vi "Get Events.vi"(11 "Create Sensor View in":refnum<class "Create Sensor View.lvclass">) -> (2 "Events":T1, 3 "Create Sensor View out":refnum<class "Create Sensor View.lvclass">)   [LabVIEW 2013, in "Create Sensor View.lvlib" / "Create Sensor View.lvclass"]
uses:
  Create Sensor View.lvclass
  Typedef/Events.ctl
  Create Sensor View.lvclass/Create Sensor View.ctl
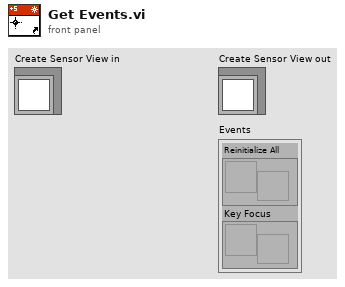
[diagram p1: front panel]
types:
  T1 = typedef "Create Sensor View.lvlib/Create Sensor View.lvclass/Events.ctl" = cluster{"Reinitialize All":refnum<user-event>, "Key Focus":refnum<user-event>}
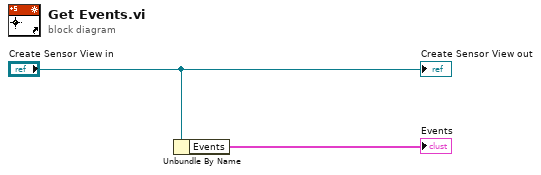
[diagram p0: block diagram]
diagram:
  n1 = Unbundle By Name("Create Sensor View in") -> ("Events"=→"Events":T1)
  "Create Sensor View out" <- "Create Sensor View in"
